vi "Choreo_DifferentialSample_Unpack.vi"(9 "StartByte":i32, 11 "RawData":u8[](array[numeric])) -> (1 "NextByte":i32, 3 "ChoreoDifferentialSample":T1={"timestamp"=-999.0, "x"=0.0, "y"=0.0, "heading"=0.0, "velocityL"=0.0, "velocityR"=0.0, "angularVelocity"=0.0, "accelL"=0.0, "accelR"=0.0, "accelAngular"=0.0, "forceL"=0.0, "forceR"=0.0})   [LabVIEW 2019, in "ChoreoLib.lvlib"]
doc: "Unpack a binary byte stream into a Differential Trajectory Sample.\n\nInputs:\n -- RawData - Byte Array - Input byte stream\n -- StartByte - Integer - Starting byte (0 relative) to parse\n\nOutputsL:\n -- ChoreoDifferentialSample - cluster - Differential trajectory sample data\n -- NextByte - integer - Index into next byte to parse"
uses:
  ChoreoLib.lvlib
  TypeDef/ChoreoDifferentialSample.ctl
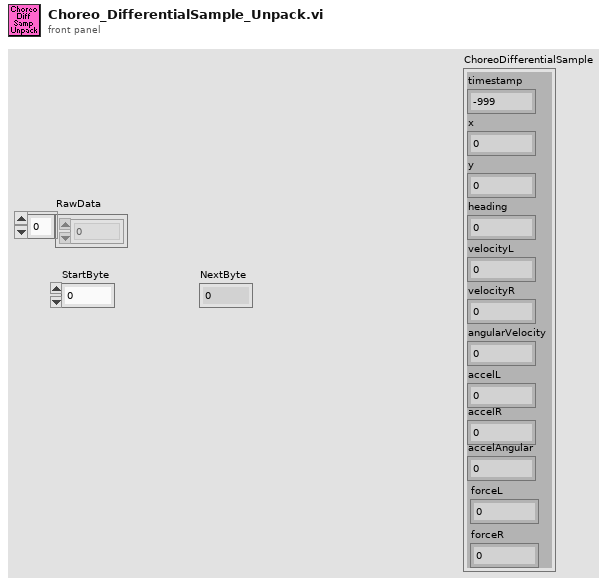
[diagram p1: front panel]
types:
  T1 = typedef "ChoreoLib.lvlib/ChoreoDifferentialSample.ctl" = cluster{"timestamp":dbl, "x":dbl, "y":dbl, "heading":dbl, "velocityL":dbl, "velocityR":dbl, "angularVelocity":dbl, "accelL":dbl, "accelR":dbl, "accelAngular":dbl, "forceL":dbl, "forceR":dbl}
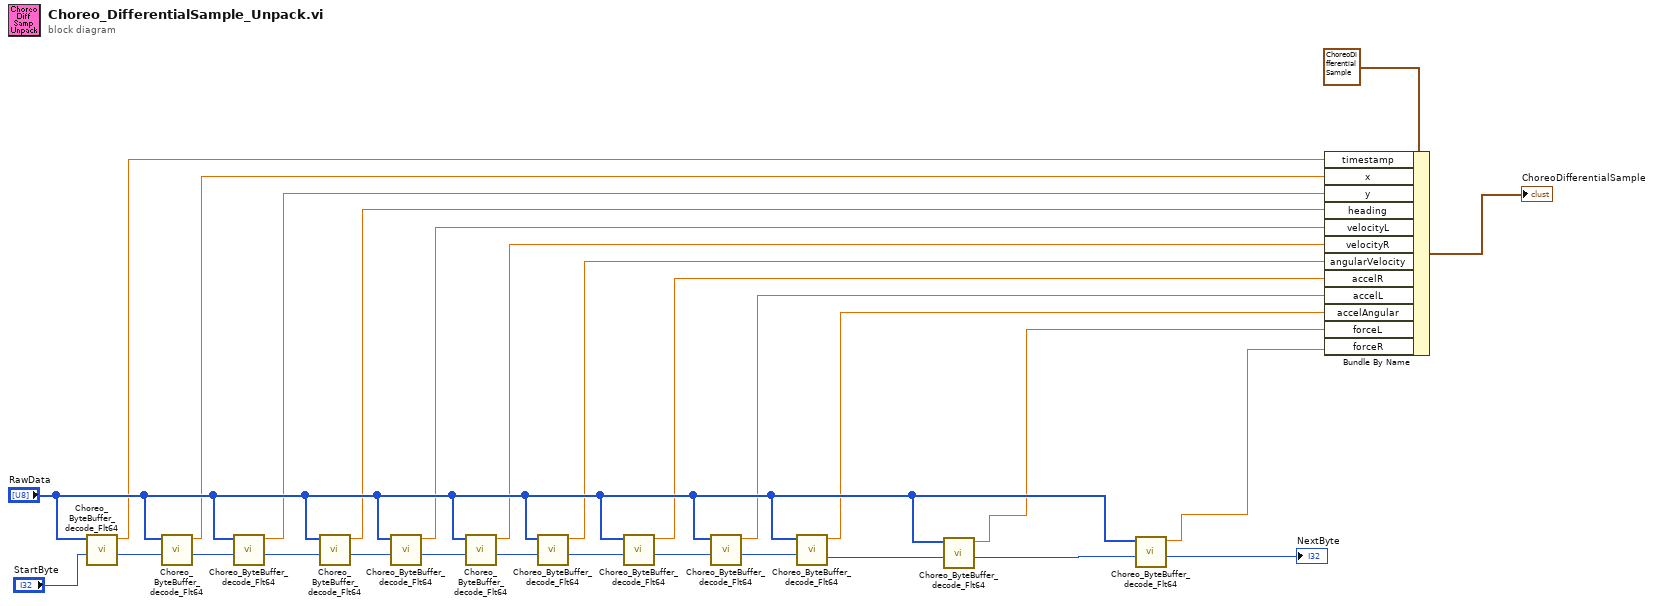
[diagram p0: block diagram]
diagram:
  n1 = call "Choreo_ByteBuffer_decode_Flt64.vi"("StartByte"="StartByte", "RawData"="RawData") -> ("NextByte"=w25:i32, "Flt64_Value"=w7:dbl)  [unwired: 8 in]
  n2 = call "Choreo_ByteBuffer_decode_Flt64.vi"("StartByte"=w25, "RawData"="RawData") -> ("NextByte"=w24:i32, "Flt64_Value"=w6:dbl)  [unwired: 8 in]
  n3 = call "Choreo_ByteBuffer_decode_Flt64.vi"("StartByte"=w24, "RawData"="RawData") -> ("NextByte"=w23:i32, "Flt64_Value"=w5:dbl)  [unwired: 8 in]
  n4 = call "Choreo_ByteBuffer_decode_Flt64.vi"("StartByte"=w23, "RawData"="RawData") -> ("NextByte"=w22:i32, "Flt64_Value"=w4:dbl)  [unwired: 8 in]
  n5 = call "Choreo_ByteBuffer_decode_Flt64.vi"("StartByte"=w22, "RawData"="RawData") -> ("NextByte"=w21:i32, "Flt64_Value"=w3:dbl)  [unwired: 8 in]
  n6 = call "Choreo_ByteBuffer_decode_Flt64.vi"("StartByte"=w21, "RawData"="RawData") -> ("NextByte"=w20:i32, "Flt64_Value"=w2:dbl)  [unwired: 8 in]
  n7 = call "Choreo_ByteBuffer_decode_Flt64.vi"("StartByte"=w20, "RawData"="RawData") -> ("NextByte"=w19:i32, "Flt64_Value"=w8:dbl)  [unwired: 8 in]
  n8 = call "Choreo_ByteBuffer_decode_Flt64.vi"("StartByte"=w19, "RawData"="RawData") -> ("NextByte"=w18:i32, "Flt64_Value"=w9:dbl)  [unwired: 8 in]
  n9 = call "Choreo_ByteBuffer_decode_Flt64.vi"("StartByte"=w18, "RawData"="RawData") -> ("NextByte"=w17:i32, "Flt64_Value"=w10:dbl)  [unwired: 8 in]
  n10 = call "Choreo_ByteBuffer_decode_Flt64.vi"("StartByte"=w17, "RawData"="RawData") -> ("NextByte"=w16:i32, "Flt64_Value"=w11:dbl)  [unwired: 8 in]
  n11 = call "Choreo_ByteBuffer_decode_Flt64.vi"("StartByte"=w16, "RawData"="RawData") -> ("NextByte"=w14:i32, "Flt64_Value"=w12:dbl)  [unwired: 8 in]
  n12 = call "Choreo_ByteBuffer_decode_Flt64.vi"("StartByte"=w14, "RawData"="RawData") -> ("NextByte"=→"NextByte":i32, "Flt64_Value"=w13:dbl)  [unwired: 8 in]
  n13 = Bundle By Name(cluster=T1 {"timestamp"=-999.0, "x"=0.0, "y"=0.0, "heading"=0.0, "velocityL"=0.0, "velocityR"=0.0, "angularVelocity"=0.0, "accelL"=0.0, "accelR"=0.0, "accelAngular"=0.0, "forceL"=0.0, "forceR"=0.0} ("ChoreoSwerveSample"), "timestamp"=w7, "x"=w6, "y"=w5, "heading"=w4, "velocityL"=w3, "velocityR"=w2, "angularVelocity"=w8, "accelR"=w9, "accelL"=w10, "accelAngular"=w11, "forceL"=w12, "forceR"=w13) -> (→"ChoreoDifferentialSample":T1)
